vi "GV-CursorHmove.vi"(7 "Gviewer in":refnum<class "Gviewer.lvclass">, 8 "error in (no error)":errorcluster, 9 "New coordinate":T1, 10 "Pos":cluster{"x":i16, "y":i16}, 11 "pict in":picture) -> (0 "error out":errorcluster, 3 "pict out":picture, 5 "Gviewer out":refnum<class "Gviewer.lvclass">)   [LabVIEW 2020, in "Sgraph_lib_V1.lvlib" / "Gviewer.lvclass"]
doc: "Andre Koelewijn, 14 feb 2021\n\nTime hand move cursor draw"
uses:
  Gviewer.lvclass
  <vilib>/Utility/miscctls.llb/LVPoint32TypeDef.ctl
  Gviewer.lvclass/Gviewer.ctl
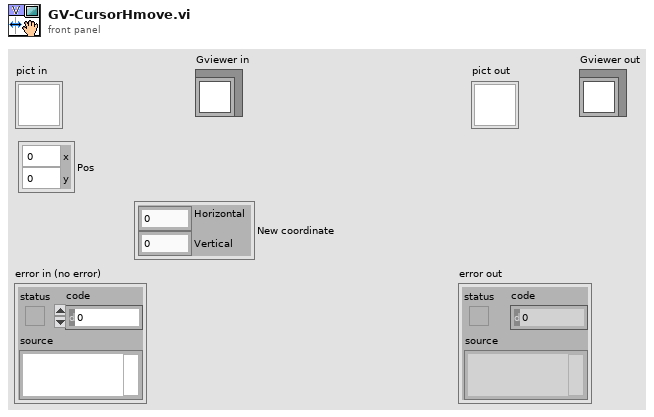
[diagram p1: front panel]
types:
  T1 = typedef "LVPoint32TypeDef.ctl" = cluster{"Horizontal":i32, "Vertical":i32}
  T2 = cluster{"horizontal":enum16{"left", "center", "right"}, "vertical":enum16{"top", "center", "bottom"}}
  T3 = cluster{"Width":u16, "Style":enum32{"Solid", "Dash", "Dot", "DashDot", "DashDotDot"}}
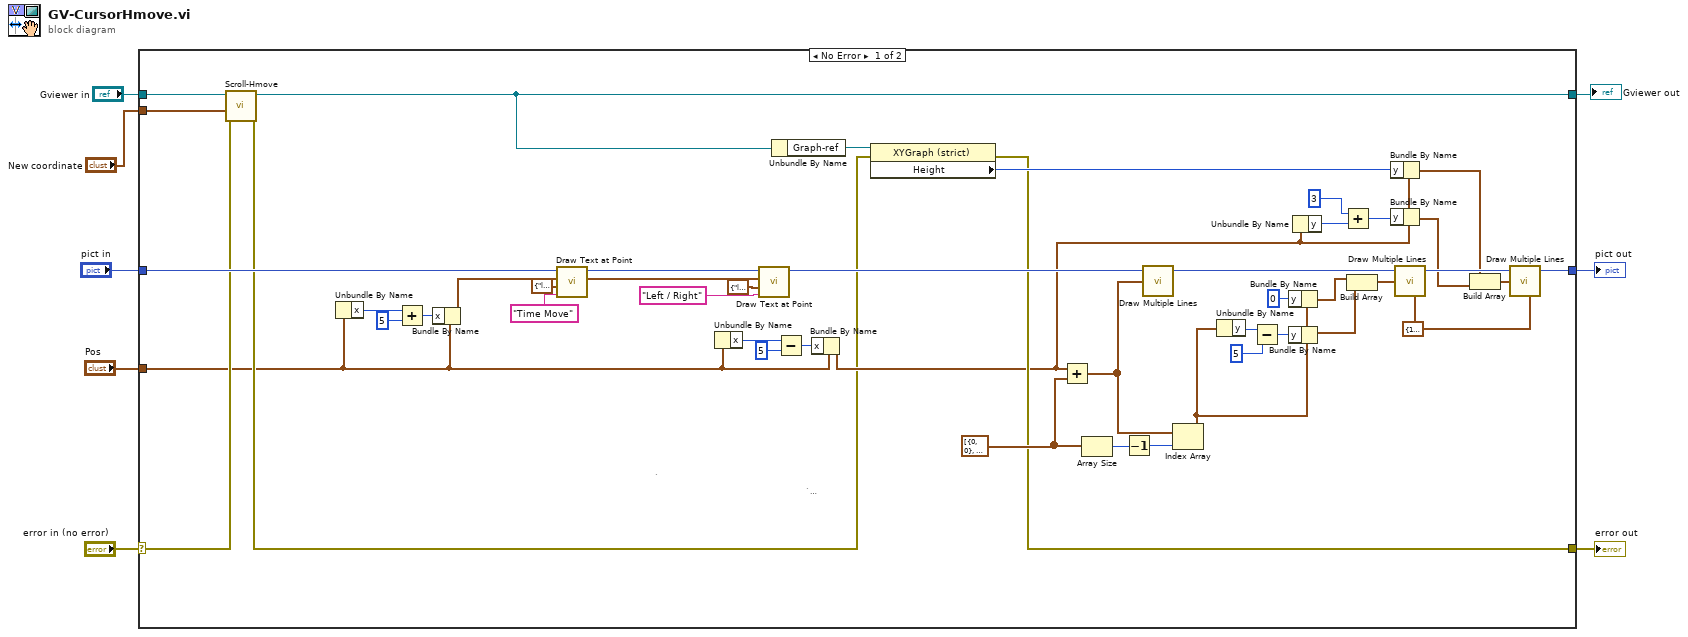
[diagram p0: block diagram]
diagram:
  n1 = case shown="No Error" "error in (no error)" {
    selector: "error in (no error)" -> [w16 w57]
    tunnel: [w20 w57] -> w7
    tunnel: "pict in" -> [w30 w56]
    tunnel: [w39 w56] -> w5
    tunnel: "Pos" -> [w10 _]
    tunnel: "Gviewer in" -> [w18 w55]
    tunnel: "New coordinate" -> [w17 _]
    tunnel: [w9 w55] -> w1
    frame No Error {
      w48 = T3 {"Width"=1, "Style"=enum."Dash"} ("pen")
      w53 = cluster{"x":i16, "y":i16}[] [{"x"=0, "y"=0}, {"x"=0, "y"=-20}, {"x"=10, "y"=-20}, {"x"=10, "y"=-15}, {"x"=20, "y"=-25}, {"x"=10, "y"=-35}, {"x"=10, "y"=-30}, {"x"=-10, "y"=-30}, {"x"=-10, "y"=-25}, {"x"=-20, "y"=-35}, {"x"=-10, "y"=-45}, {"x"=-10, "y"=-40}, {"x"=0, "y"=-40}, {"x"=0, "y"=-50}] ("line endpoints")
      # "`"
      # "``"
      n2 = call "Scroll-Hmove.vi"("error in (no error)"=w16, "New coordinate"=w17, "Gviewer in"=w18) -> ("error out"=w15:errorcluster, "Gviewer out"=w9:refnum<class "Gviewer.lvclass">)  [unwired: 7 in]
      n3 = Unbundle By Name(w10) -> ("x"=w12:i16)
      n4 = Add(x=w12, y=i16 5) -> (x+y=w14:i16)
      n5 = Bundle By Name(cluster=w10, "x"=w14) -> (w11:cluster{"x":i16, "y":i16})
      n6 = call <vilib>:"Draw Text at Point.vi"("text"="Time Move", "alignment(left, top)"=T2 {"horizontal"=enum."left", "vertical"=enum."bottom"}, "origin"=w11, "picture"=w30) -> ("new picture"=w27:picture)  [unwired: 6 in, 1 out]
      n7 = Unbundle By Name(w10) -> ("x"=w26:i16)
      n8 = call <vilib>:"Draw Text at Point.vi"("text"="Left / Right", "alignment(left, top)"=T2 {"horizontal"=enum."left", "vertical"=enum."top"}, "origin"=w11, "picture"=w27) -> ("new picture"=w23:picture)  [unwired: 6 in, 1 out]
      n9 = Unbundle By Name(w9) -> ("Graph-ref"=w22:refnum<vi>)
      n10 = Subtract(x=w26, y=i16 5) -> (x-y=w24:i16)
      n11 = Bundle By Name(cluster=w10, "x"=w24) -> (w19:cluster{"x":i16, "y":i16})
      n12 = property class="XYGraph (strict)"(reference=w22, error in=w15) -> (error out=w20:errorcluster, "Height"=w21:u32)  [unwired: 1 out]
      n13 = Add(x=w19, y=w53) -> (x+y=w50:cluster{"x":i16, "y":i16}[])
      n14 = Array Size(array=w53) -> (size(s)=w52:i32)
      n15 = Decrement(x=w52) -> (x-1=w51:i32)
      n16 = call <vilib>:"Draw Multiple Lines.vi"("picture"=w23, "line endpoints"=w50) -> ("new picture"=w54:picture)  [unwired: 7 in]
      n17 = Index Array(array=w50, index=w51) -> (element=w42:cluster{"x":i16, "y":i16})
      n18 = Unbundle By Name(w42) -> ("y"=w47:i16)
      n19 = Subtract(x=w47, y=i16 5) -> (x-y=w45:i16)
      n20 = Bundle By Name(cluster=w42, "y"=i16 0 ("x")) -> (w41:cluster{"x":i16, "y":i16})
      n21 = Bundle By Name(cluster=w42, "y"=w45) -> (w44:cluster{"x":i16, "y":i16})
      n22 = Unbundle By Name(w19) -> ("y"=w38:i16)
      n23 = Add(x=i16 3, y=w38) -> (x+y=w37:i16)
      n24 = Build Array(w41, w44) -> (w49:cluster{"x":i16, "y":i16}[])
      n25 = Bundle By Name(cluster=w19, "y"=w21) -> (w33:cluster{"x":i16, "y":i16})
      n26 = Bundle By Name(cluster=w19, "y"=w37) -> (w34:cluster{"x":i16, "y":i16})
      n27 = call <vilib>:"Draw Multiple Lines.vi"("picture"=w54, "line endpoints"=w49, "pen"=w48) -> ("new picture"=w40:picture)  [unwired: 6 in]
      n28 = Build Array(w33, w34) -> (w35:cluster{"x":i16, "y":i16}[])
      n29 = call <vilib>:"Draw Multiple Lines.vi"("picture"=w40, "line endpoints"=w35, "pen"=w48) -> ("new picture"=w39:picture)  [unwired: 6 in]
    }
    frame Error {
    }
  }
  "error out" <- w7
  "pict out" <- w5
  "Gviewer out" <- w1
